vi "TCM1021_sendcmd.vi"(0 "com in":refnum<visa-resource-name>, 1 "command in":u8[](array[numeric]), 2 "错误输入":errorcluster caption="错误输入（无错误）") -> (3 "com out":refnum<visa-resource-name>, 4 "dataout":i32, 5 "return out":u8[](array[numeric]), 6 "错误输出":errorcluster)   [LabVIEW 2018]
panel:
  out "return out 2":u8[](array[numeric])
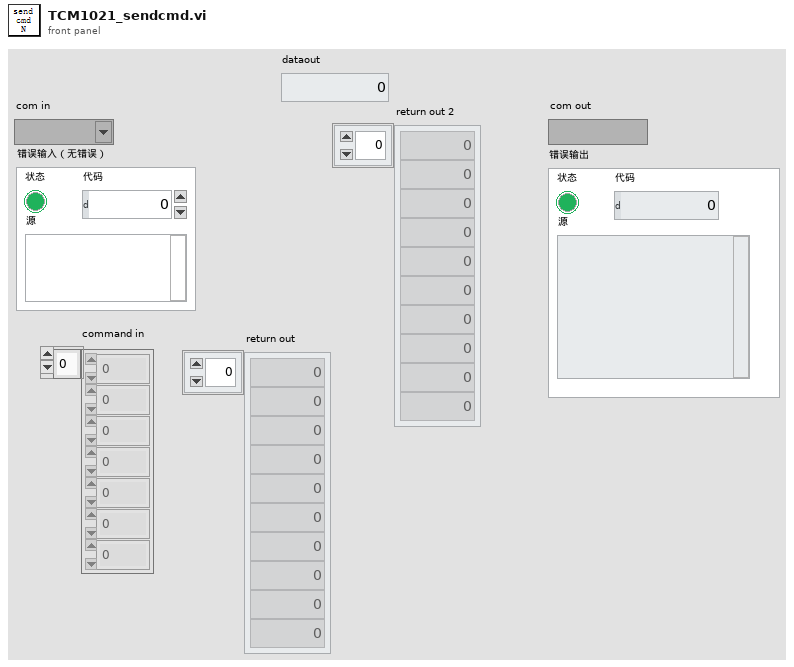
[diagram p1: front panel]
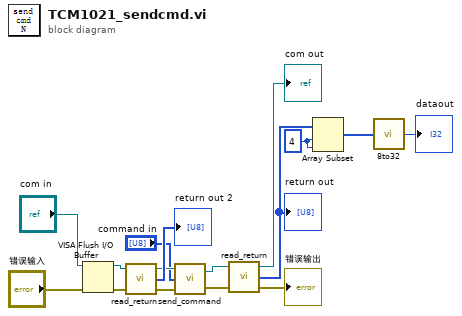
[diagram p0: block diagram]
diagram:
  w14 = 4 ("索引")
  n1 = VISA Flush I/O Buffer(VISA resource name="com in", error in (no error)="错误输入") -> (VISA resource name out=w11:refnum<visa-resource-name>, error out=w10:errorcluster)  [unwired: 1 in]
  n2 = call "read_return.vi"("错误输入（无错误）"=w10, "com in"=w11) -> ("错误输出"=w3:errorcluster, "return out"=→"return out 2":u8[], "com out"=w5:refnum<visa-resource-name>)  [unwired: 1 in]
  n3 = call "send_command.vi"("错误输入"=w3, 3:"command in", "com in"=w5) -> ("错误输出"=w1:errorcluster, "com out"=w2:refnum<visa-resource-name>)
  n4 = call "read_return.vi"("错误输入（无错误）"=w1, "com in"=w2) -> ("错误输出"=→"错误输出":errorcluster, "return out"=w7:u8[], "com out"=→"com out":refnum<visa-resource-name>)  [unwired: 1 in]
  "return out" <- w7
  n5 = Array Subset(array=w7, index=w14, length=w14) -> (w13:u8[])
  n6 = call "8to32.vi"("Arrayin"=w13) -> ("data32"=→"dataout":i32)
